vi "PPG_ABC.convert temp pattern to string arrays.vi"(0 "i ref in":refnum<vi>, 2 "patternDefs":T1(array[cluster]), 4 "clockRate [ticks/us]":dbl, 5 "error in (no error)":errorcluster) -> (14 "i ref out":refnum<vi>, 16 "patternArray":string[](array[string]), 19 "error out":errorcluster)   [LabVIEW 2014, in "PPG_ABC.lvlib"]
doc: "Converts the intermediate pattern format to a format that is specific to the parent class."
uses:
  PPG_ABC.lvlib
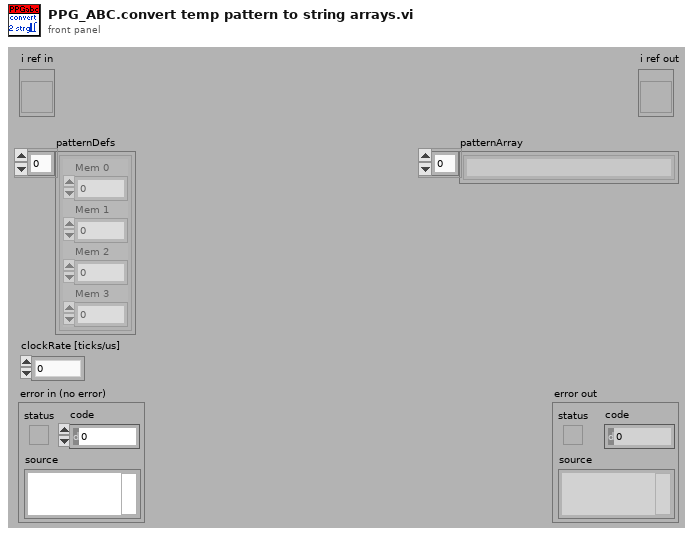
[diagram p1: front panel]
types:
  T1 = cluster{"Mem 0":u8, "Mem 1":u32, "Mem 2":u32, "Mem 3":u32}[]
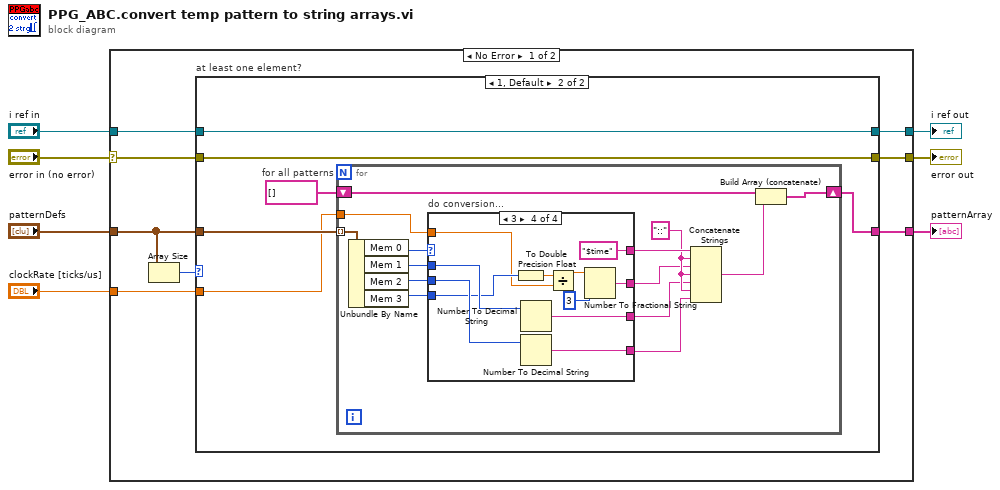
[diagram p0: block diagram]
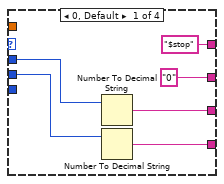
[diagram p3: hidden frame]
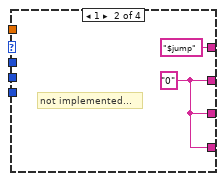
[diagram p4: hidden frame]
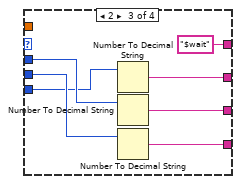
[diagram p5: hidden frame]
diagram:
  n1 = case shown="No Error" "error in (no error)" {
    selector: "error in (no error)" -> [w12 w64]
    tunnel: "i ref in" -> [w14 w65]
    tunnel: [w13 w65] -> w6
    tunnel: [w11 w64] -> w5
    tunnel: "patternDefs" -> [w10 _]
    tunnel: [w9 _] -> w2
    tunnel: "clockRate [ticks/us]" -> [w8 _]
    frame No Error {
      n2 = Array Size(array=w10) -> (size(s)=w15:i32)
      n3 = case "at least one element?" shown="1, Default" w15 {
        tunnel: [w17 w19] -> w13
        tunnel: w14 -> [w17 w19]
        tunnel: w12 -> [w16 w20]
        tunnel: [w16 w20] -> w11
        tunnel: w10 -> [_ w23]
        tunnel: [_ w21] -> w9
        tunnel: w8 -> [_ w18]
        frame 0 {
        }
        frame 1, Default {
          n4 = for "for all patterns" {
            tunnel: w23 -> [w37] mode=indexing
            shift-right: [w26] -> w21
            shift-left: string[] [] -> [w28]
            tunnel: w18 -> [w24]
            w32 = "::" ("string")
            n5 = Unbundle By Name(w37) -> ("Mem 0"=w36:u8, "Mem 1"=w35:u32, "Mem 2"=w34:u32, "Mem 3"=w25:u32)
            n6 = case "do conversion..." shown="3" w36 {
              tunnel: ["$stop" "$jump" "$wait" "$time"] -> w33
              tunnel: w35 -> [w42 _ w51 w62]
              tunnel: [w41 w44 w50 w61] -> w30
              tunnel: w34 -> [w40 _ w49 w60]
              tunnel: [w39 w44 w48 w59] -> w29
              tunnel: ["0" w44 w47 w58] -> w31
              tunnel: w25 -> [_ _ w46 w57]
              tunnel: w24 -> [_ _ _ w53]
              frame 0, Default {
                n7 = Number To Decimal String(number=w42) -> (decimal integer string=w41:string)  [unwired: 1 in]
                n8 = Number To Decimal String(number=w40) -> (decimal integer string=w39:string)  [unwired: 1 in]
              }
              frame 1 {
                w44 = "0"
                # "not implemented..."
              }
              frame 2 {
                n9 = Number To Decimal String(number=w46) -> (decimal integer string=w47:string)  [unwired: 1 in]
                n10 = Number To Decimal String(number=w51) -> (decimal integer string=w50:string)  [unwired: 1 in]
                n11 = Number To Decimal String(number=w49) -> (decimal integer string=w48:string)  [unwired: 1 in]
              }
              frame 3 {
                n12 = To Double Precision Float(number=w57) -> (double precision float=w56:dbl)
                n13 = Number To Decimal String(number=w62) -> (decimal integer string=w61:string)  [unwired: 1 in]
                n14 = Number To Decimal String(number=w60) -> (decimal integer string=w59:string)  [unwired: 1 in]
                n15 = Divide(x=w56, y=w53) -> (x/y=w55:dbl)
                n16 = Number To Fractional String(number=w55, precision (6)=i16 3) -> (F-format string=w58:string)  [unwired: 2 in]
              }
            }
            n17 = Concatenate Strings(w33, w32, w31, w32, w30, w32, w29) -> (w27:string)
            n18 = Build Array (concatenate)(w28, w27) -> (w26:string[])
          }
        }
      }
    }
    frame Error {
    }
  }
  "error out" <- w5
  "i ref out" <- w6
  "patternArray" <- w2
